vi "Set RFPM Present.vi"(0 "TSM Context In":T1, 5 "RFPM Present":bool, 11 "error in":errorcluster) -> (4 "TSM Context Out":T1, 15 "error out":errorcluster)   [LabVIEW 2023, in "RFFixtureCharact.RFPM.lvlib" / "RF Subsystem Session Provider.lvclass"]
uses:
  RF Subsystem Session Provider.lvclass
  <vilib>/NI_TestStand_SemiconductorModule/NI_TestStand_Semiconductor_Module.lvlibp/PinMap/General/SemiconductorModuleContext.ctl
  Common/RF Subsystem Session Provider/Utilities/Global Data Id Prefix.vi
  <vilib>/NI_TestStand_SemiconductorModule/NI_TestStand_Semiconductor_Module.lvlibp
  Common/RFCalAndFixtureCharact.Common.lvlib
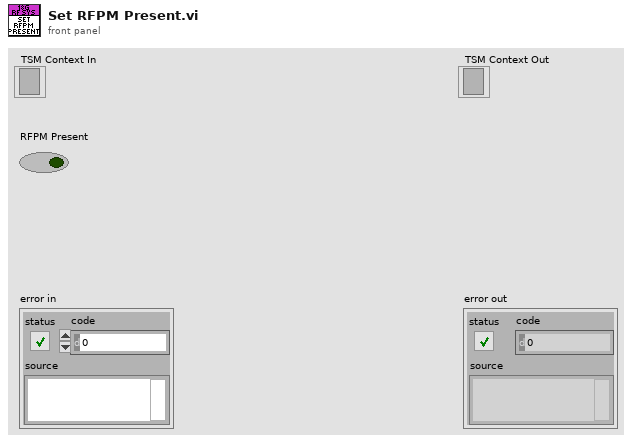
[diagram p1: front panel]
types:
  T1 = typedef "NI_TestStand_Semiconductor_Module.lvlibp/SemiconductorModuleContext.ctl" = refnum<k7>
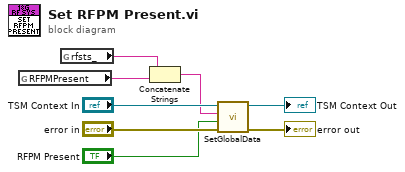
[diagram p0: block diagram]
diagram:
  n1 = global read "Global Data Id Prefix.vi" "RFPMPresent"() -> (w2:string)
  n2 = global read "Global Data Id Prefix.vi" "rfsts_"() -> (w3:string)
  n3 = Concatenate Strings(w3, w2) -> (w1:string)
  n4 = call <vilib>:"SetGlobalData.vi"("error in (no error)"="error in", "Data"="RFPM Present", "Data Id"=w1, "Semiconductor Module Context"="TSM Context In") -> ("error out"=→"error out":errorcluster, "Semiconductor Module Context Out"=→"TSM Context Out":T1)  [unwired: 5 in]
